vi "Acnet XML-RPC Multi-Device Reader.vi"(8 "error in (no error)":errorcluster, 11 "Devices":string[](array[string])) -> (0 "error out":errorcluster, 3 "Readings":T1(array[cluster]))   [LabVIEW 2013]
uses:
  <vilib>/httpClient/POSTBuffer.vi
  <vilib>/httpClient/LabVIEWHTTPClient.lvlib
panel:
  out "headers":string
  out "body":string
  in  "url":string="www-bd.fnal.gov/xmlrpc/Accelerator"
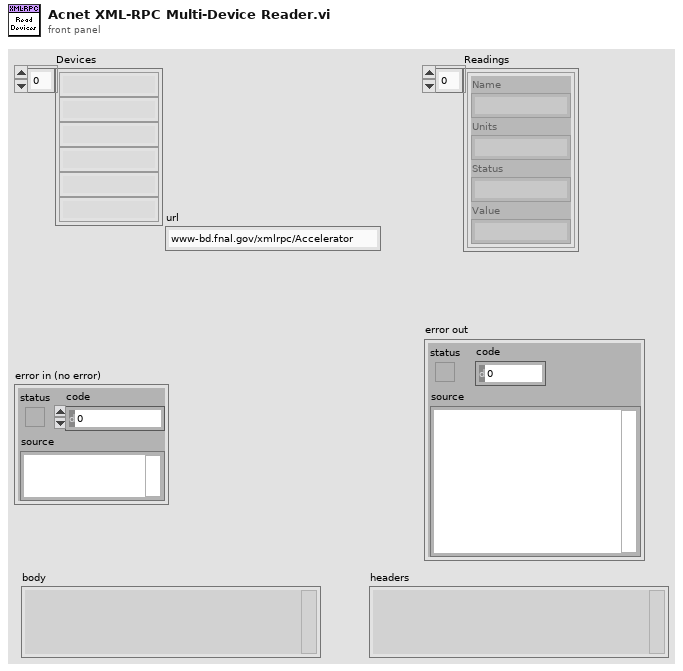
[diagram p1: front panel]
types:
  T1 = cluster{"Name":string, "Units":string, "Status":string, "Value":string}[]
  T2 = typedef "LabVIEWHTTPClient.lvlib/ClientHandle.ctl" = refnum<k1>
  T3 = cluster{"Name":string, "Units":string, "Status":string, "Value":string}
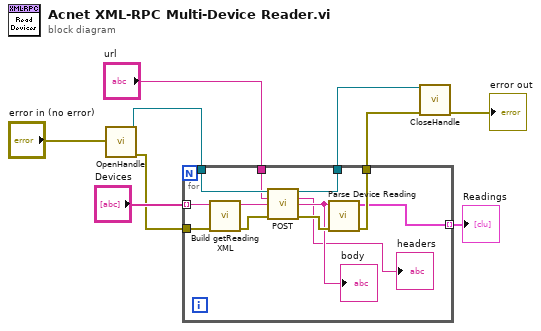
[diagram p0: block diagram]
diagram:
  n1 = call <vilib>:"OpenHandle.vi"("error in (no error)"="error in (no error)") -> ("client handle out"=w8:T2, "error out"=w4:errorcluster)  [unwired: 13 in]
  n2 = for {
    tunnel: [w21] -> w9
    tunnel: w8 -> [w20]
    tunnel: "url" -> [w19]
    tunnel: "Devices" -> [w17] mode=indexing
    tunnel: w4 -> [w16]
    tunnel: [w13] -> w3
    tunnel: [w12] -> w1 mode=indexing
    n3 = call "Build getReading XML.vi"("error in (no error)"=w16, "Device"=w17) -> ("error out"=w15:errorcluster, "XML"=w18:string)  [unwired: 8 in]
    n4 = call-poly <vilib>:"POST.vi"("client handle"=w20, "url"=w19, "buffer"=w18, "error in (no error)"=w15) -> ("client handle out"=w21:T2, "headers"=→"headers":string, "body"=w11:string, "error out"=w14:errorcluster)  [unwired: 8 in]
    "body" <- w11
    n5 = call "Parse Device Reading.vi"("error in (no error)"=w14, "Reading XML"=w11) -> ("error out"=w13:errorcluster, "Reading"=w12:T3)  [unwired: 8 in]
  }
  "Readings" <- w1
  n6 = call <vilib>:"CloseHandle.vi"("client handle"=w9, "error in (no error)"=w3) -> ("error out"=→"error out":errorcluster)  [unwired: 13 in]
